vi "ContinueScan.vi"(8 "error in":errorcluster, 9 "Instrument":string="KIM", 10 "Scan Cluster":T1={"Scanning Segments Left"=0, "Path"=path "", "FileName"="", "Scan Segments"=0, "Step Time (us)"=100, "Polarity"=enum."Positive", "Direction"=enum."Forward", "Steps"=1, "Acq per step"=1} {"Acq per step" min=1 max=10000 step=1 scale=1.0..10000.0; "Steps" min=1 max=10000 step=1 scale=1.0..10000.0; "Step Time (us)" min=100 step=10 scale=100.0..10000.0; "Scan Segments" max=100 step=1 scale=0.0..100.0}, 11 "Message Enqueuer in":refnum<class "Message Enqueuer.lvclass">) -> (0 "error out":errorcluster, 2 "Scan Cluster":T1={"Scanning Segments Left"=0, "Path"=path "", "FileName"="", "Scan Segments"=0, "Step Time (us)"=100, "Polarity"=enum."Positive", "Direction"=enum."Forward", "Steps"=1, "Acq per step"=1} {"Acq per step" min=1 max=10000 step=1 scale=1.0..10000.0; "Steps" min=1 max=10000 step=1 scale=1.0..10000.0; "Step Time (us)" min=100 step=10 scale=100.0..10000.0; "Scan Segments" max=100 step=1 scale=0.0..100.0})   [LabVIEW 2023, in "InterferometryUI.lvlib" / "InterferometryUI.lvclass"]
uses:
  InterferometryUI.lvclass
  Libraries/KIM101_Actor/KIM101/KIM101 Messages/MoveBySteps Msg/MoveBySteps Msg.lvclass
  Libraries/SinglePhotonInterferenceUI/SinglePhotonInterferenceUI Messages/MH_Ext_Acquire Msg/MH_Ext_Acquire Msg.lvclass
  <vilib>/ActorFramework/Message Enqueuer/Message Enqueuer.lvclass
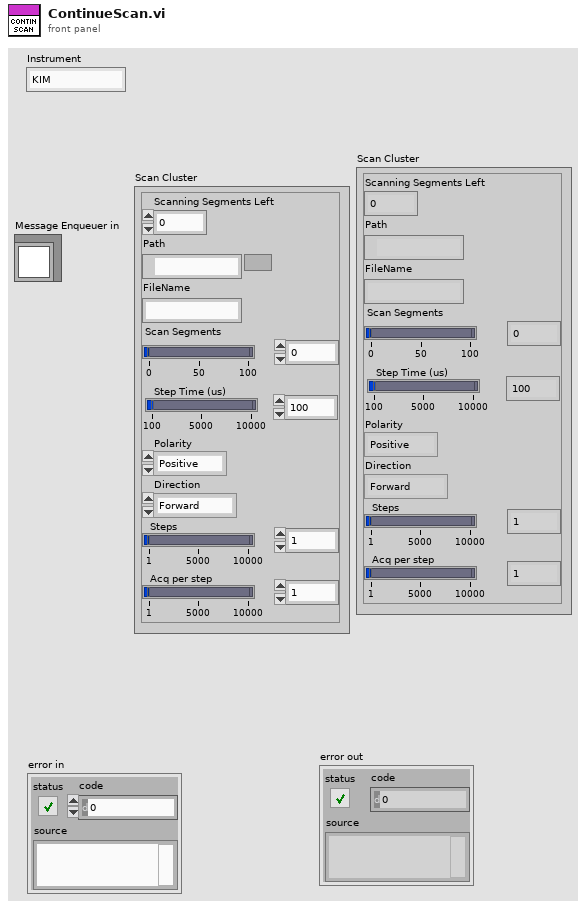
[diagram p1: front panel]
types:
  T1 = cluster{"Scanning Segments Left":u16, "Path":path, "FileName":string, "Scan Segments":u32, "Step Time (us)":u32, "Polarity":enum16{"Positive", "Negative"}, "Direction":enum16{"Forward", "Backwards"}, "Steps":u32, "Acq per step":u32}
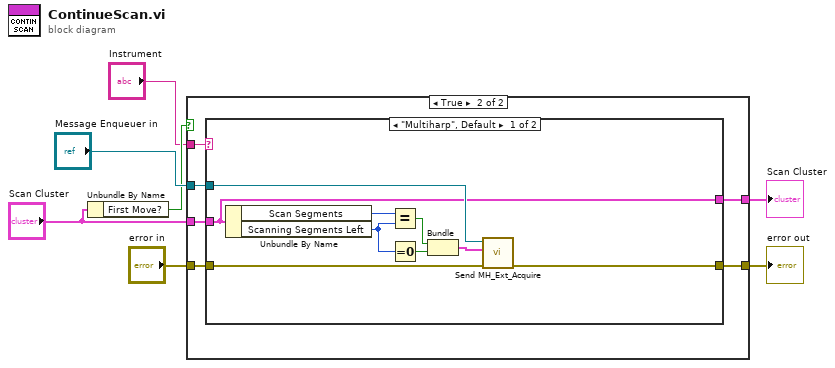
[diagram p0: block diagram]
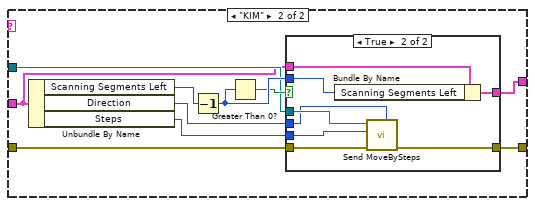
[diagram p3: hidden frame]
diagram:
  n1 = Unbundle By Name("Scan Cluster") -> ("First Move?"=w6:bool)
  n2 = case shown="True" w6 {
    tunnel: [w9 w15] -> w4
    tunnel: "Message Enqueuer in" -> [_ w14]
    tunnel: "Scan Cluster" -> [w9 w13]
    tunnel: [w8 w10] -> w3
    tunnel: "error in" -> [w8 w11]
    tunnel: "Instrument" -> [_ w12]
    frame False {
    }
    frame True {
      n3 = case shown="\"Multiharp\", Default" w12 {
        tunnel: [w22 w34] -> w15
        tunnel: w14 -> [w24 w31]
        tunnel: w13 -> [w22 w29]
        tunnel: w11 -> [w21 w25]
        tunnel: [w20 w26] -> w10
        frame "Multiharp", Default {
          n4 = Unbundle By Name(w22) -> ("Scan Segments"=w19:u32, "Scanning Segments Left"=w17:u16)
          n5 = Equal?(x=w19, y=w17) -> (x = y?=w18:bool)
          n6 = Equal To 0?(x=w17) -> (x = 0?=w16:bool)
          n7 = Bundle(w18, w16) -> (w23:cluster{bool, bool})  [unwired: 1 in]
          n8 = call "Send MH_Ext_Acquire.vi"("error in (no error)"=w21, "event data"=w23, "Message Enqueuer"=w24) -> ("error out"=w20:errorcluster)  [unwired: 7 in, 1 out]
        }
        frame "KIM" {
          n9 = Unbundle By Name(w29) -> ("Scanning Segments Left"=w30:u16, "Direction"=w27:enum16{"Forward", "Backwards"}, "Steps"=w28:u32)
          n10 = Decrement(x=w30) -> (x-1=w33:u16)
          n11 = Greater Than 0?(x=w33) -> (x > 0?=w32:bool)
          n12 = case shown="True" w32 {
            tunnel: [w35 w43] -> w34
            tunnel: w33 -> [_ w44]
            tunnel: w31 -> [_ w41]
            tunnel: w29 -> [w35 w42]
            tunnel: w28 -> [_ w40]
            tunnel: w27 -> [_ w39]
            tunnel: [w36 w38] -> w26
            tunnel: w25 -> [w36 w37]
            frame False {
            }
            frame True {
              n13 = Bundle By Name(cluster=w42, "Scanning Segments Left"=w44) -> (w43:T1)
              n14 = call "Send MoveBySteps.vi"("Direction"=w39, "error in (no error)"=w37, "Steps"=w40, "Message Enqueuer"=w41) -> ("error out"=w38:errorcluster)  [unwired: 6 in, 1 out]
            }
          }
        }
      }
    }
  }
  "Scan Cluster" <- w4
  "error out" <- w3
